vi "test_top.vi"() -> ()   [LabVIEW 2025, in "LabJackEKG.lvlib"]
uses:
  LabJackEKG.lvlib
  StreamProducerLoopData.ctl
  Typedefs/AcquisitionConfig.ctl
  Typedefs/LabJackData.ctl
panel:
  out "Now":timestamp
  out "start":timestamp
  out "Read Data":T1 {"TC [degC]" format="%#_f"; "RMS [V]" format="%#_f"; "Volume [L]" format="%#_f"; "Flow [L/min]" format="%#_f"; "Spin  [RPM]" format="%#_f"}
  in  "LabJackConfig":T2={"Drum Reflectors"=4, "Drum Max. Samping Window [s]"=2.0, "Drum Min. Sampling Window [s]"=0.5, "Flow Max. Samping Window [s]"=1.0, "Flow Min. Sampling Window [s]"=0.25, "Flow mL/pulse"=[1.0, 1.0, 1.0], "Flow Offset mL"=[1.0, 1.0, 1.0], "RMS Sampling Window [s]"=3.0, "TC Sampling Window [s]"=0.25, "TC Scale"=[1.0, 1.0], "TC Offset [V]"=[0.0, 0.0]} {"TC Offset [V]" format="%#_f"; "TC Scale" format="%#_f"; "Flow Offset mL" format="%#_f"; "Flow mL/pulse" format="%#_f"}
  out "error out 2":errorcluster
  out "stop inbd":bool
  in  "error in (no error)":errorcluster
  in  "ms":u32=100
  out "error out":errorcluster={"status"=TRUE, "code"=8607, "source"="LJM_eStreamStart.vi"}
  in  "stop":bool
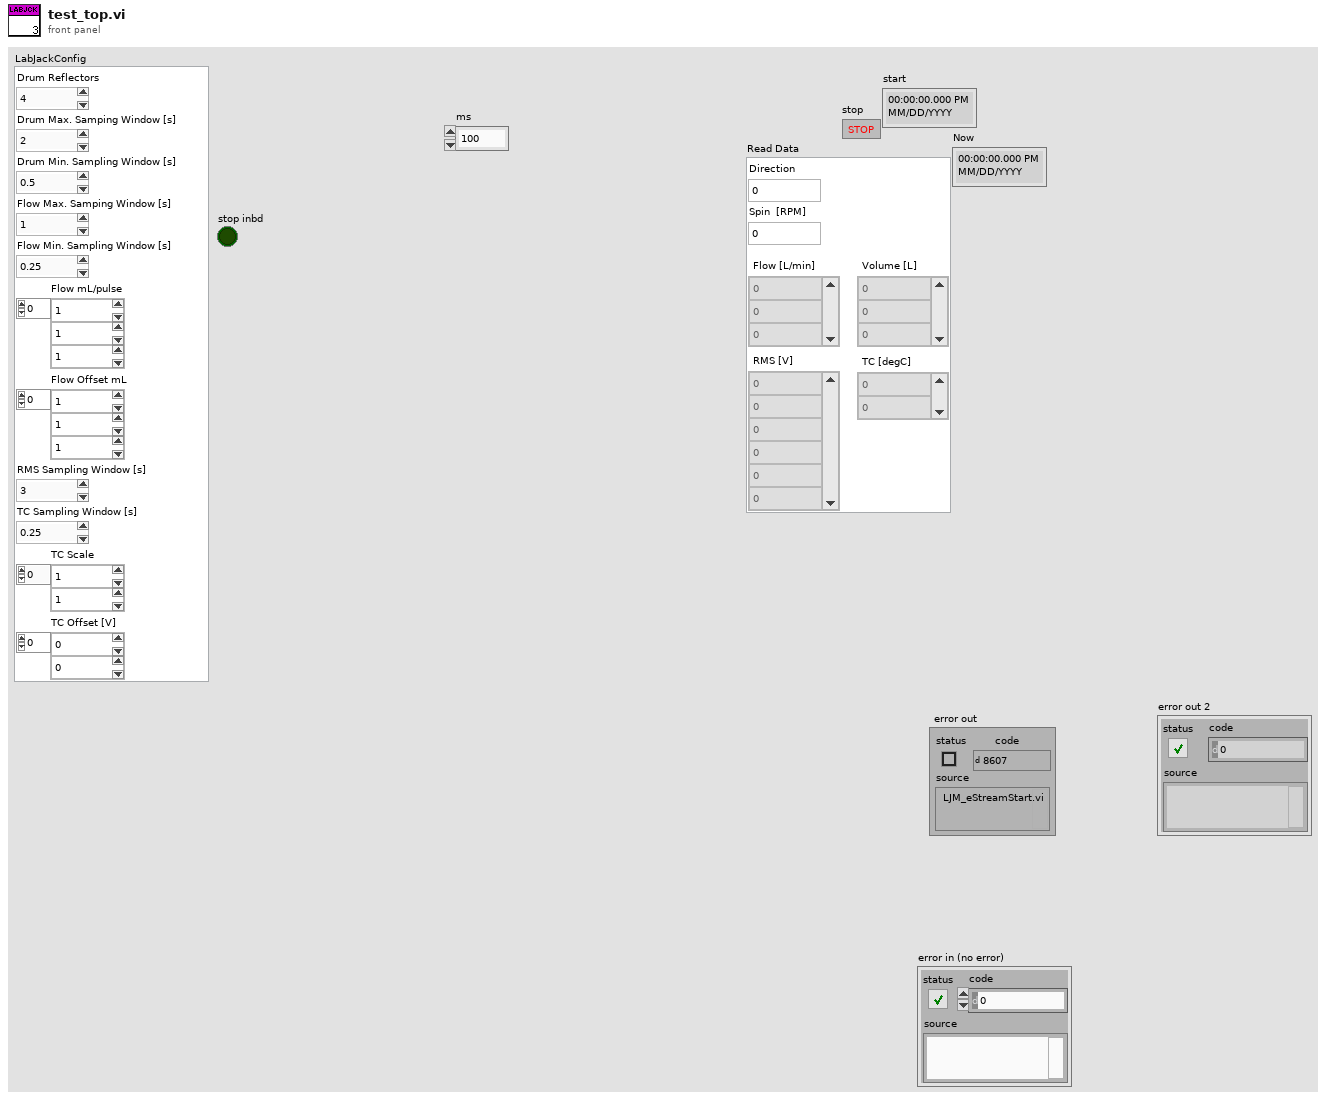
[diagram p1: front panel]
types:
  T1 = typedef "LabJackEKG.lvlib/LabJackData.ctl" = cluster{"Direction":i32, "Spin  [RPM]":dbl, "Flow [L/min]":dbl[], "Volume [L]":dbl[], "RMS [V]":dbl[], "TC [degC]":dbl[]}
  T2 = typedef "LabJackEKG.lvlib/AcquisitionConfig.ctl" = cluster{"Drum Reflectors":i64, "Drum Max. Samping Window [s]":dbl, "Drum Min. Sampling Window [s]":dbl, "Flow Max. Samping Window [s]":dbl, "Flow Min. Sampling Window [s]":dbl, "Flow mL/pulse":dbl[], "Flow Offset mL":dbl[], "RMS Sampling Window [s]":dbl, "TC Sampling Window [s]":dbl, "TC Scale":dbl[], "TC Offset [V]":dbl[]}
  T3 = typedef "LabJackEKG.lvlib/StreamProducerLoopData.ctl" = cluster{"Count":i64, "Time":i64, "Initialized":bool}
  T4 = typedef "LabJackGlobalResources.ctl" = cluster{"DIrQ":refnum<queue>, "CntQ":refnum<queue>[], "AiQ":refnum<queue>[]}
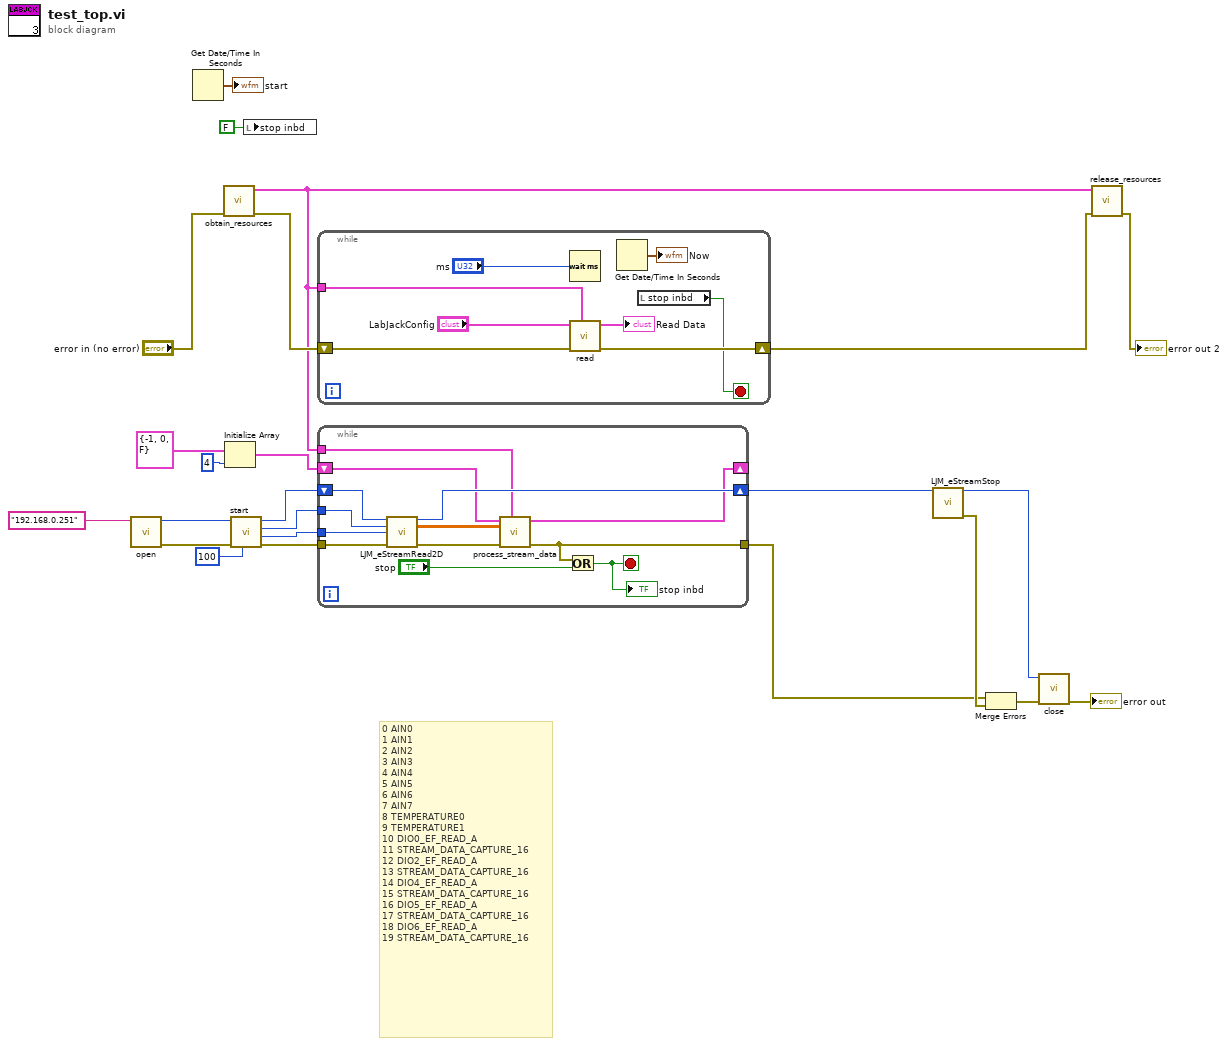
[diagram p0: block diagram]
diagram:
  # "0 AIN0\n1 AIN1\n2 AIN2\n3 AIN3\n4 AIN4\n5 AIN5\n6 AIN6\n7 AIN7\n8 TEMPERATURE0\n9 TEMPERATURE1\n10 DIO0_EF_READ_A\n11 STREAM_DATA_CAPTURE_16\n12 DIO2_EF_READ_A\n13 STREAM_DATA_CAPTURE_16\n14 DIO4_EF_READ_A\n15 STREAM_DATA_CAPTURE_16\n16 DIO5_EF_READ_A\n17 STREAM_DATA_CAPTURE_16\n18 DIO6_EF_READ_A\n19 STREAM_DATA_CAPTURE_16"
  n1 = call "open.vi"("IP Address (LJM_idANY )"="192.168.0.251") -> ("error out"=w24:errorcluster, "Handle"=w23:i32)  [unwired: 8 in, 1 out]
  n2 = Get Date/Time In Seconds() -> (seconds since 1Jan1904=→"start":timestamp)
  n3 = call "obtain_resources.vi"("error in (no error)"="error in (no error)") -> ("error out"=w9:errorcluster, "LabJackRes"=w3:T4)  [unwired: 9 in]
  n4 = Initialize Array(T3 {"Count"=-1, "Time"=0, "Initialized"=FALSE} ("output cluster"), 4 ("dimension size")) -> (w7:T3[])
  n5 = call "start.vi"("Period [ms]"=100, "error in (no error)"=w24, "Handle In"=w23) -> ("error out"=w22:errorcluster, "NumReadAddresses"=w19:i32, "ScansPerRead Out"=w20:i32, "Handle Out"=w21:i32)  [unwired: 5 in]
  n6 = local write "stop inbd"(FALSE ("stop inbd")) -> ()
  n7 = while {
    tunnel: w3 -> [w25]
    shift-right: [w32] -> w2
    shift-left: w9 -> [w31]
    stop <- w28 stop-if-true
    n8 = Wait (ms)(milliseconds to wait="ms") -> ()  [unwired: 1 out]
    n9 = call "read.vi"("Queues"=w25, "error in (no error)"=w31, "LabJackConfig"="LabJackConfig") -> ("error out"=w32:errorcluster, "Read Data"=→"Read Data":T1)  [unwired: 7 in]
    n10 = Get Date/Time In Seconds() -> (seconds since 1Jan1904=→"Now":timestamp)
    n11 = local read "stop inbd"() -> (w28:bool)
  }
  n12 = while {
    tunnel: w22 -> [w45]
    tunnel: [w38] -> w11
    tunnel: w20 -> [w43]
    tunnel: w19 -> [w44]
    shift-right: [w39] -> w15
    shift-left: w21 -> [w42]
    tunnel: w3 -> [w33]
    shift-right: [w36] -> _
    shift-left: w7 -> [w35]
    stop <- w40 stop-if-true
    n13 = call <vilib>:"LJM_eStreamRead2D.vi"("Handle In"=w42, "ScansPerRead"=w43, "NumAddresses"=w44, "error in"=w45) -> ("Handle Out"=w39:i32, "aData Out"=w34:dbl[][], "error out"=w37:errorcluster)  [unwired: 7 in, 2 out]
    n14 = call "process_stream_data.vi"("Queues"=w33, "error in (no error)"=w37, "aData Out"=w34, "Loop Data In"=w35) -> ("error out"=w38:errorcluster, "Loop Data Out"=w36:T3[])  [unwired: 6 in]
    n15 = Or(x=w38, y="stop") -> (x .or. y?=w40:bool)
    "stop inbd" <- w40
  }
  n16 = call <vilib>:"LJM_eStreamStop.vi"("Handle In"=w15) -> ("Handle Out"=w14:i32, "error out"=w12:errorcluster)  [unwired: 13 in]
  n17 = Merge Errors(w11, w12) -> (w13:errorcluster)
  n18 = call "close.vi"("error in"=w13, "Handle"=w14) -> ("error out"=→"error out":errorcluster)  [unwired: 9 in]
  n19 = call "release_resources.vi"("error in (no error)"=w2, "LabJackRes"=w3) -> ("error out"=→"error out 2":errorcluster)  [unwired: 9 in]
